vi "Loop_PDP_SEN.vi"() -> ()   [LabVIEW 2017, in "System_Status.lvlib"]
uses:
  System_Status.lvlib
  TypeDef Share All/CLUSTER_PDP_Status.ctl
  TypeDef Share All/CLUSTER_PDP_Faults.ctl
  CLUSTER_System_CMD.ctl
  Global Share All/Global_STOP.vi
  Global_CMD.vi
  Global_SEN Write_Data.vi
panel:
  in  "PDP ID":i32
  out "Cycle Time (S)":dbl format="%.3g"
  in  "Target Time(ms)":u32=50
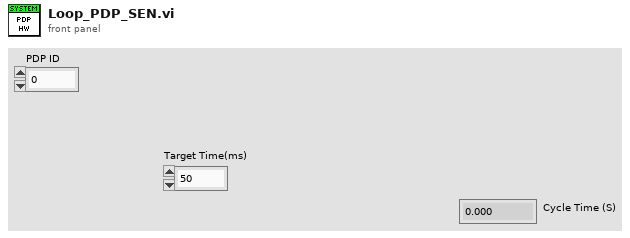
[diagram p1: front panel]
types:
  T1 = typedef "System_Status.lvlib/CLUSTER_System_CMD.ctl" = cluster{"Enable PCM Monitoring":bool, "Enable PDP Monitoring":bool, "Enable RoboRio Monitoring":bool}
  T2 = typedef "CLUSTER_PDP_Status.ctl" = cluster{"PDP Faults":T3, "All Currents (A)":dbl[], "Energy (J)":dbl, "Power (W)":dbl, "Voltage (V)":dbl}
  T3 = typedef "CLUSTER_PDP_Faults.ctl" = cluster{"Current Faults":bool[], "Batt V Fault":bool, "Temp Fault":bool, "HW Fault":bool}
  T4 = cluster{"PDP ID":i32, "Target Time(ms)":u32, "Current Time":timestamp, "Previous Time":timestamp, "Cycle Time (S)":dbl, "PDP Status":T2, "Enabled":T1}
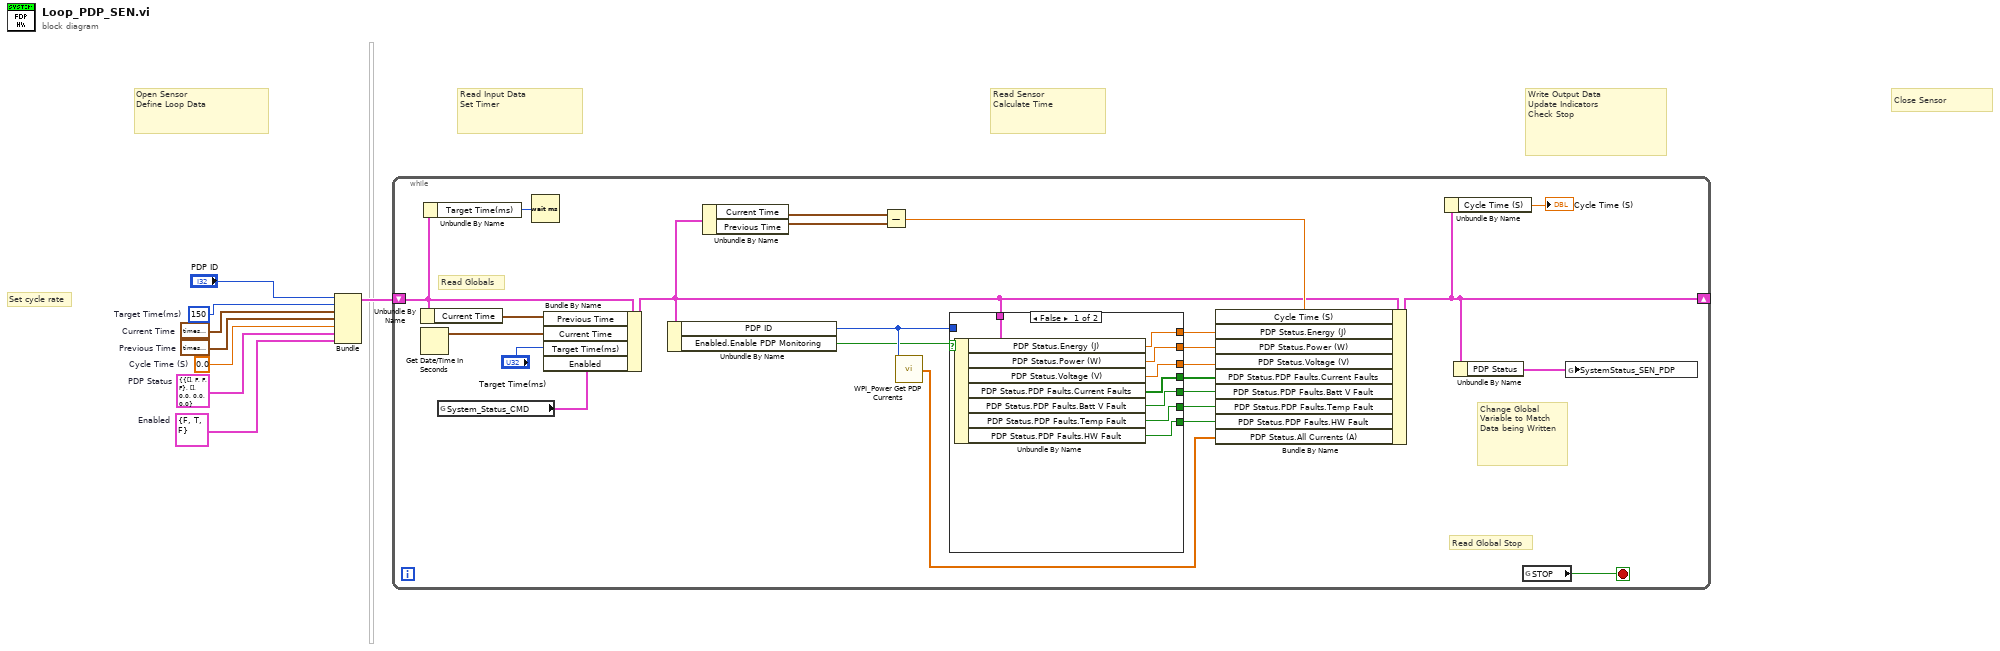
[diagram p0: block diagram]
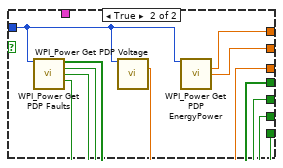
[diagram p2: hidden frame]
diagram:
  w1 = T1 {"Enable PCM Monitoring"=FALSE, "Enable PDP Monitoring"=TRUE, "Enable RoboRio Monitoring"=FALSE}  # Enabled
  w2 = T2 {"PDP Faults"={"Current Faults"=[], "Batt V Fault"=FALSE, "Temp Fault"=FALSE, "HW Fault"=FALSE}, "All Currents (A)"=[], "Energy (J)"=0.0, "Power (W)"=0.0, "Voltage (V)"=0.0}  # PDP Status
  w4 = 0.0  # Cycle Time (S)
  w8 = timestamp(0 s since 1904-01-01)  # Previous Time
  w7 = timestamp(0 s since 1904-01-01)  # Current Time
  w6 = u32 150  # Target Time(ms)
  # "Close Sensor"
  # "Write Output Data\nUpdate Indicators\nCheck Stop"
  # "Read Sensor\nCalculate Time"
  # "Read Input Data\nSet Timer"
  # "Open Sensor\nDefine Loop Data"
  # "Set cycle rate"
  n1 = Bundle("PDP ID"="PDP ID", "Target Time(ms)"=w6, "Current Time"=w7, "Previous Time"=w8, "Cycle Time (S)"=w4, "PDP Status"=w2, "Enabled"=w1) -> (w5:T4)  [unwired: 1 in]
  n2 = while {
    shift-right: [w23] -> _
    shift-left: w5 -> [w25]
    stop <- w32 stop-if-true
    # "Change Global\nVariable to Match\nData being Written"
    # "Read Globals"
    # "Read Global Stop"
    n3 = Unbundle By Name(w25) -> ("Current Time"=w29:timestamp)
    n4 = Get Date/Time In Seconds() -> (seconds since 1Jan1904=w30:timestamp)
    n5 = Unbundle By Name(w25) -> ("Target Time(ms)"=w24:u32)
    n6 = global read "Global_CMD.vi" "System_Status_CMD"() -> (w11:T1)
    n7 = Wait (ms)(milliseconds to wait=w24) -> ()  [unwired: 1 out]
    n8 = Bundle By Name(cluster=w25, "Previous Time"=w29, "Current Time"=w30, "Target Time(ms)"="Target Time(ms)", "Enabled"=w11) -> (w9:T4)
    n9 = Unbundle By Name(w9) -> ("PDP ID"=w20:i32, "Enabled.Enable PDP Monitoring"=w10:bool)
    n10 = Unbundle By Name(w9) -> ("Current Time"=w28:timestamp, "Previous Time"=w27:timestamp)
    n11 = Subtract(x=w28, y=w27) -> (x-y=w21:dbl)
    n12 = call <vilib>:"WPI_Power Get PDP Currents.vi"("Power Distribution Panel (0)"=w20) -> ("all currents (A)"=w19:dbl[])  [unwired: 12 in, 2 out]
    n13 = case shown="False" w10 {
      tunnel: w20 -> [_ w48]
      tunnel: [w36 w47] -> w18
      tunnel: [w35 w46] -> w17
      tunnel: [w34 w45] -> w16
      tunnel: [w33 w44] -> w15
      tunnel: [w37 w43] -> w14
      tunnel: [w38 w42] -> w13
      tunnel: [w39 w41] -> w12
      tunnel: w9 -> [w40 _]
      frame False {
        n14 = Unbundle By Name(w40) -> ("PDP Status.Energy (J)"=w39:dbl, "PDP Status.Power (W)"=w38:dbl, "PDP Status.Voltage (V)"=w37:dbl, "PDP Status.PDP Faults.Current Faults"=w36:bool[], "PDP Status.PDP Faults.Batt V Fault"=w35:bool, "PDP Status.PDP Faults.Temp Fault"=w34:bool, "PDP Status.PDP Faults.HW Fault"=w33:bool)
      }
      frame True {
        n15 = call <vilib>:"WPI_Power Get PDP Faults.vi"("Power Distribution Panel (0)"=w48) -> ("Current Faults"=w47:bool[], "Battery Voltage Fault"=w46:bool, "Temperature Fault"=w45:bool, "Hardware Fault"=w44:bool)  [unwired: 10 in, 1 out]
        n16 = call <vilib>:"WPI_Power Get PDP Voltage.vi"("Power Distribution Panel (0)"=w48) -> ("voltage (V)"=w43:dbl)  [unwired: 13 in, 1 out]
        n17 = call <vilib>:"WPI_Power Get PDP EnergyPower.vi"("Power Distribution Panel (0)"=w48) -> ("Energy (J)"=w41:dbl, "Power (W)"=w42:dbl)  [unwired: 12 in, 1 out]
      }
    }
    n18 = Bundle By Name(cluster=w9, "Cycle Time (S)"=w21, "PDP Status.Energy (J)"=w12, "PDP Status.Power (W)"=w13, "PDP Status.Voltage (V)"=w14, "PDP Status.PDP Faults.Current Faults"=w18, "PDP Status.PDP Faults.Batt V Fault"=w17, "PDP Status.PDP Faults.Temp Fault"=w16, "PDP Status.PDP Faults.HW Fault"=w15, "PDP Status.All Currents (A)"=w19) -> (w23:T4)
    n19 = Unbundle By Name(w23) -> ("Cycle Time (S)"=→"Cycle Time (S)":dbl)
    n20 = Unbundle By Name(w23) -> ("PDP Status"=w31:T2)
    n21 = global read "Global_STOP.vi" "STOP"() -> (w32:bool)
    n22 = global write "Global_SEN Write_Data.vi" "SystemStatus_SEN_PDP"(w31) -> ()
  }
